vi "Configure Pulse Limit.vi"(8 "error in (no error)":errorcluster, 9 "Limit":dbl, 10 "Function (0:Voltage)":u16(ring) items=["Voltage", "Current"], 11 "VISA resource name":refnum<visa-resource-name>="USB0::0x05E6::0x2461::04090176::INSTR") -> (0 "error out":errorcluster, 3 "VISA resource name out":refnum<visa-resource-name>)   [LabVIEW 2017, in "Keithley 2450.lvlib"]
doc: "This command sets the source limit for pulse outputs. The Model 2461 cannot source pulse levels\nthat exceed this limit.\n\nWhen the function set is Voltage, the limit applies to Current.\nWhen the function set is Current, the limit applies to Voltage.\n\nThe values that can be set for this command are limited by the setting for the overvoltage protection\nlimit. Also, if an interlock is not installed, the values are limited.\nThis value can also be limited by the measurement range. If a specific measurement range is set, the\nlimit must be more than 1 percent of the measurement range. If you set the measurement range to be\nautomatically selected, the measurement range is selected based on the pulse and bias limits.\nIf you change the source range to a level that is not appropriate for this limit, the instrument changes\nthe source limit to a limit that is appropriate to the range and a warning is generated.\nLimits are absolute values.\n\n<B>This function is only compatible with the 2461.</B>"
uses:
  Keithley 2450.lvlib
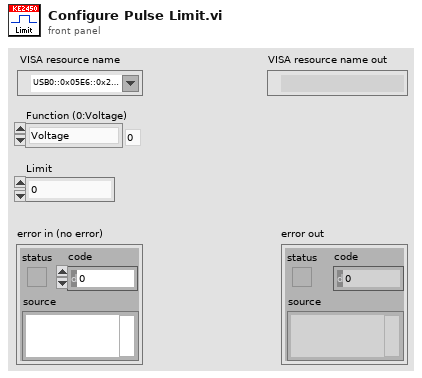
[diagram p1: front panel]
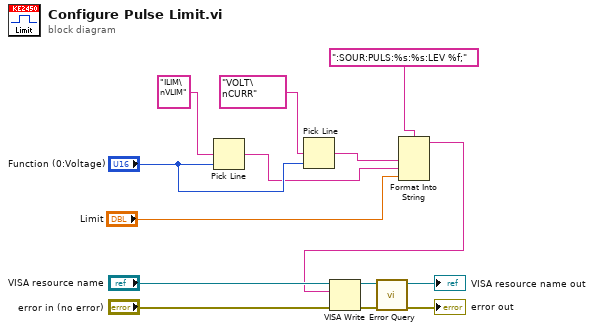
[diagram p0: block diagram]
diagram:
  n1 = Pick Line(multi-line string="ILIM\nVLIM", line index="Function (0:Voltage)") -> (output string=w6:string)  [unwired: 1 in]
  n2 = Pick Line(multi-line string="VOLT\nCURR", line index="Function (0:Voltage)") -> (output string=w5:string)  [unwired: 1 in]
  n3 = Format Into String(format string=":SOUR:PULS:%s:%s:LEV %f;" ("multi-line string"), w5, w6, "Limit") -> (resulting string=w1:string)  [unwired: 2 in, 1 out]
  n4 = VISA Write(VISA resource name="VISA resource name", write buffer=w1, error in (no error)="error in (no error)") -> (VISA resource name out=w10:refnum<visa-resource-name>, error out=w9:errorcluster)  [unwired: 1 out]
  n5 = call "Error Query.vi"("error in (no error)"=w9, "VISA resource name"=w10) -> ("error out"=→"error out":errorcluster, "VISA resource name out"=→"VISA resource name out":refnum<visa-resource-name>)  [unwired: 8 out]
